vi "Read BLRL Config.vi"(8 "error in (no error)":errorcluster, 11 "BluelinesRedlines Source in":refnum<class "BluelinesRedlines Source.lvclass">) -> (0 "error out":errorcluster, 2 "BLRL Config":T1, 3 "BluelinesRedlines Source out":refnum<class "BluelinesRedlines Source.lvclass">)   [LabVIEW 2020, in "VolatusGUI.lvlib" / "BluelinesRedlines Source.lvclass"]
uses:
  BluelinesRedlines Source.lvclass
  BLRL Config.ctl
  Range Limit Config.ctl
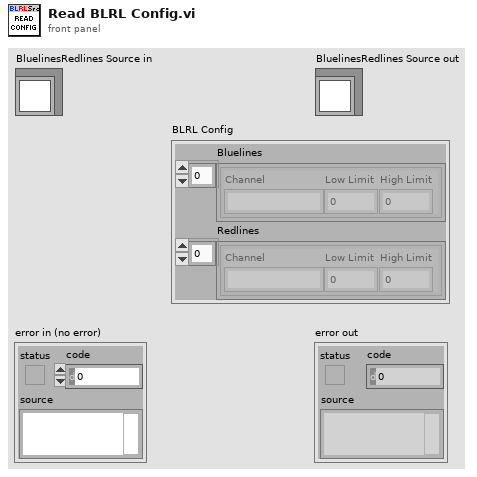
[diagram p1: front panel]
types:
  T1 = typedef "VolatusGUI.lvlib/BluelinesRedlines Source.lvclass/BLRL Config.ctl" = cluster{"Bluelines":T2[], "Redlines":T2[]}
  T2 = typedef "VolatusGUI.lvlib/BluelinesRedlines Source.lvclass/Range Limit Config.ctl" = cluster{"Channel":string, "Low Limit":dbl, "High Limit":dbl}
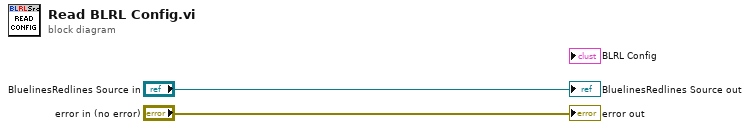
[diagram p0: block diagram]
diagram:
  "error out" <- "error in (no error)"
  "BluelinesRedlines Source out" <- "BluelinesRedlines Source in"
